vi "Serial_TEST (1).vi"() -> ()   [LabVIEW 2019]
uses:
  Program Files (x86)/National Instruments/LabVIEW 2019/examples/Instrument IO/Serial/support/Serial - Settings.ctl
  <vilib>/Instr/_visa.llb/VISA Configure Serial Port (Instr).vi
panel:
  out "mode":u8
  out "unsigned byte array[0]":u8
  out "Waveform Chart":T1(graph)
  in  "Termination Character":u8=10 format="%.0x"
  in  "VISA resource name":refnum<visa-resource-name>="COM1"
  in  "Serial Settings":T2={"baud rate"=9600, "data bits"=8, "parity"=enum."None", "stop bits"=10, "flow control"=0} {"flow control" items=["None"=0, "XON/XOFF"=1, "RTS/CTS"=2, "DTR/DSR"=4]; "stop bits" items=["1.0"=10, "1.5"=15, "2.0"=20]; "data bits" min=5 max=8 step=1; "baud rate" items=["75"=75, "110"=110, "134"=134, "150"=150, "300"=300, "600"=600, "1200"=1200, "1800"=1800, "2400"=2400, "4800"=4800, "7200"=7200, "1"=9600, "14400"=14400, "19200"=19200, "28800"=28800, "38400"=38400, "56000"=56000, "57600"=57600, "115200"=115200, "128000"=128000, "230400"=230400]}
  in  "End Read on Termination Character?":bool=TRUE
  out "read buffer":string
  in  "write buffer":string
  in  "stop":bool
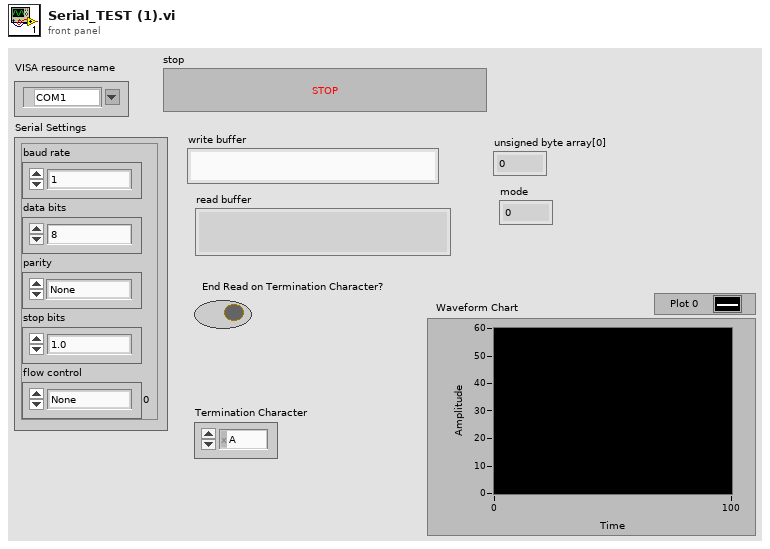
[diagram p1: front panel]
types:
  T1 = cluster{"unsigned byte array[0]":u8, "unsigned byte array[1]":u8, "unsigned byte array[2]":u8, "unsigned byte array[3]":u8, "unsigned byte array[4]":u8, "unsigned byte array[5]":u8, "unsigned byte array[6]":u8, "unsigned byte array[7]":u8, "unsigned byte array[8]":u8}
  T2 = typedef "Serial - Settings.ctl" = cluster{"baud rate":u32, "data bits":u16, "parity":enum16{"None", "Odd", "Even", "Mark", "Space"}, "stop bits":u16, "flow control":u16}
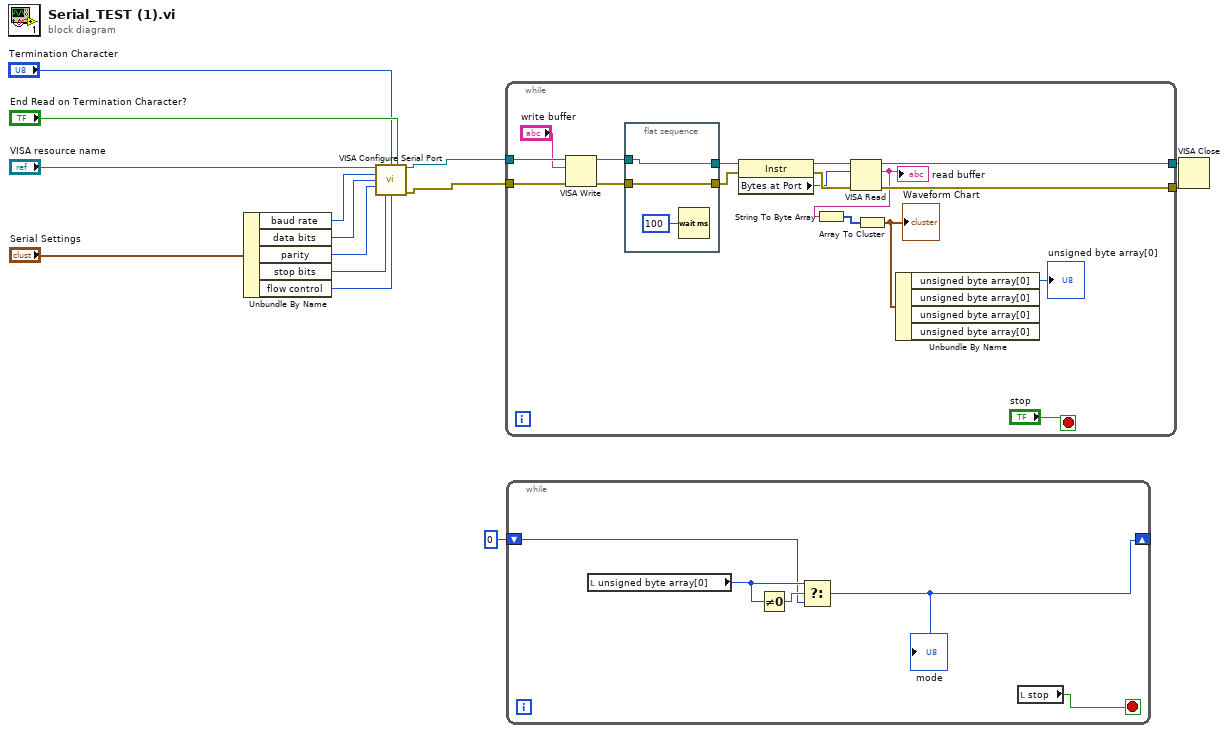
[diagram p0: block diagram]
diagram:
  n1 = Unbundle By Name("Serial Settings") -> ("baud rate"=w8:u32, "data bits"=w9:u16, "parity"=w10:enum16{"None", "Odd", "Even", "Mark", "Space"}, "stop bits"=w11:u16, "flow control"=w5:u16)
  n2 = call-poly "VISA Configure Serial Port"("VISA resource name"="VISA resource name", "termination char\n(0xA = '\\n' = LF)"="Termination Character", "Enable Termination\nChar (T)"="End Read on Termination Character?", "baud rate (9600)"=w8, "data bits (8)"=w9, "parity (0:none)"=w10, "stop bits (10: 1 bit)"=w11, "flow control (0:none)"=w5) -> ("VISA resource name out"=w3:refnum<visa-resource-name>, "error out"=w2:errorcluster)  [unwired: 2 in, 4 out]
  n3 = while {
    tunnel: w3 -> [w30]
    tunnel: [w29] -> w14
    tunnel: w2 -> [w28]
    tunnel: [w27] -> w13
    stop <- "stop" stop-if-true
    n4 = VISA Write(VISA resource name=w30, write buffer="write buffer", error in (no error)=w28) -> (VISA resource name out=w25:refnum<visa-resource-name>, error out=w24:errorcluster)  [unwired: 1 out]
    n5 = flat-sequence {
      tunnel: w25 -> [w32]
      tunnel: w24 -> [w34]
      tunnel: [w34] -> w21
      tunnel: [w32] -> w23
      frame #0 {
        n6 = Wait (ms)(milliseconds to wait=u32 100) -> ()  [unwired: 1 out]
      }
    }
    n7 = property class="Instr"(reference=w23, error in=w21) -> (reference out=w22:refnum<visa-resource-name>, error out=w20:errorcluster, "Bytes at Port"=w19:u32)
    n8 = VISA Read(VISA resource name=w22, byte count=w19, error in (no error)=w20) -> (VISA resource name out=w29:refnum<visa-resource-name>, read buffer=w18:string, error out=w27:errorcluster)  [unwired: 1 out]
    "read buffer" <- w18
    n9 = String To Byte Array(string=w18) -> (unsigned byte array=w17:u8[])
    n10 = Array To Cluster(array=w17) -> (cluster=w16:T1)
    "Waveform Chart" <- w16
    n11 = Unbundle By Name(w16) -> ("unsigned byte array[0]"=→"unsigned byte array[0]":u8)  [unwired: 3 out]
  }
  n12 = while {
    shift-right: [w35] -> _
    shift-left: u8 0 ("unsigned byte array[0]") -> [w36]
    stop <- w39 stop-if-true
    n13 = local read "unsigned byte array[0]"() -> (w38:u8)
    n14 = Not Equal To 0?(x=w38) -> (x != 0?=w37:bool)
    n15 = Select(t=w38, s=w37, f=w36) -> (s? t:f=w35:u8)
    "mode" <- w35
    n16 = local read "stop"() -> (w39:bool)
  }
  n17 = VISA Close(VISA resource name=w14, error in (no error)=w13) -> ()  [unwired: 1 out]
